vi "Lock.vi"(8 "error in (no error)":errorcluster, 11 "Timed Door in":refnum<class "Timed Door.lvclass">) -> (0 "error out":errorcluster, 3 "Timed Door out":refnum<class "Timed Door.lvclass">)   [LabVIEW 2018, in "Timed Door.lvclass"]
uses:
  Timed Door.lvclass
  Timed Door.lvclass/Timed Door.ctl
  Get Alarm DVR.vi
  Door/Door.lvclass
  Alarm/Alarm.lvclass
  Timer/Timer.lvclass
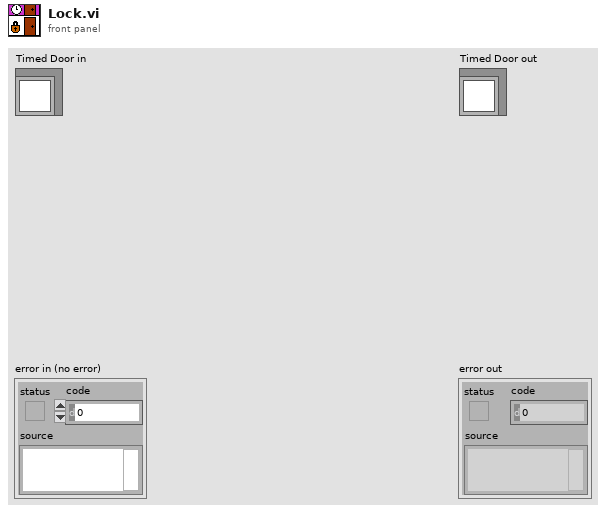
[diagram p1: front panel]
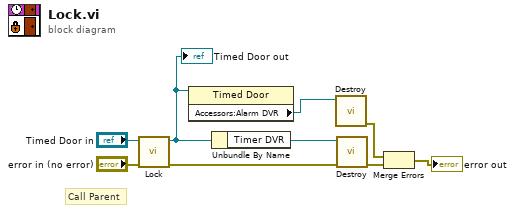
[diagram p0: block diagram]
diagram:
  # "Call Parent"
  n1 = call-parent "Lock.vi"("error in (no error)"="error in (no error)", "Door in"="Timed Door in") -> ("error out"=w7:errorcluster, "Door out"=w4:refnum<class "Timed Door.lvclass">)  [unwired: 8 in]
  "Timed Door out" <- w4
  n2 = property class="Timed Door"(reference=w4) -> ("Accessors:Alarm DVR"=w3:refnum<data-value>)  [unwired: 1 in, 2 out]
  n3 = Unbundle By Name(w4) -> ("Timer DVR"=w5:refnum<data-value>)
  n4 = call "Destroy.vi"("Alarm DVR"=w3) -> ("error out"=w1:errorcluster)  [unwired: 10 in]
  n5 = call "Destroy.vi"("error in (no error)"=w7, "Timer DVR"=w5) -> ("error out"=w6:errorcluster)  [unwired: 9 in]
  n6 = Merge Errors(w1, w6) -> (→"error out":errorcluster)
